vi "Write Driver Config.vi"(8 "error in (no error)":errorcluster, 10 "Driver Config":T1={"Joystick"=refnum, "Forward Drive"=refnum, "Sideways Drive"=refnum, "Percent Forward"=1.0, "Percent Sideways"=1.0}, 11 "Driver in":refnum<class "Driver.lvclass">) -> (0 "error out":errorcluster, 3 "Driver out":refnum<class "Driver.lvclass">)   [LabVIEW 2014, in "Driver.lvlib" / "Driver.lvclass"]
uses:
  Driver.lvclass
  Driver Config.ctl
  Joystick/Joystick Class/Joystick.lvclass
  <vilib>/ActorFramework/Message Enqueuer/Message Enqueuer.lvclass
  Driver.lvclass/Driver.ctl
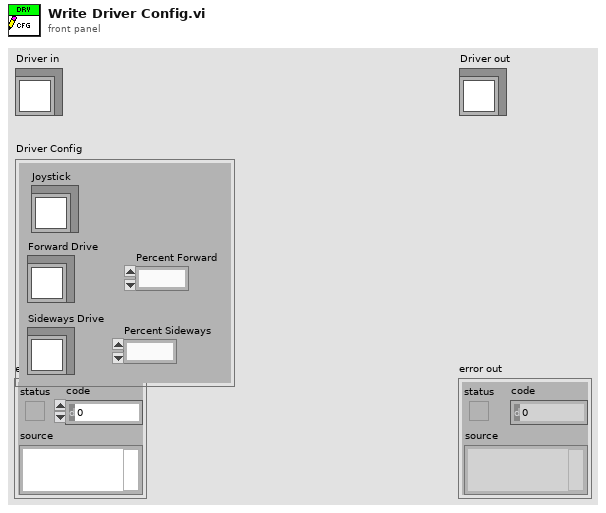
[diagram p1: front panel]
types:
  T1 = typedef "Driver.lvlib/Driver.lvclass/Driver Config.ctl" = cluster{"Joystick":refnum<class "Joystick.lvclass">, "Forward Drive":refnum<class "Message Enqueuer.lvclass">, "Sideways Drive":refnum<class "Message Enqueuer.lvclass">, "Percent Forward":dbl, "Percent Sideways":dbl}
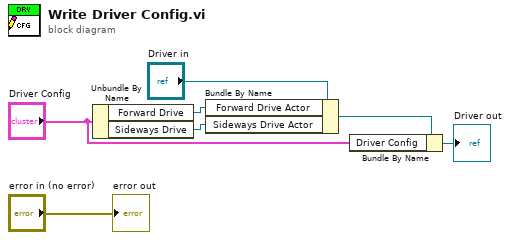
[diagram p0: block diagram]
diagram:
  n1 = Unbundle By Name("Driver Config") -> ("Forward Drive"=w2:refnum<class "Message Enqueuer.lvclass">, "Sideways Drive"=w1:refnum<class "Message Enqueuer.lvclass">)
  n2 = Bundle By Name(cluster="Driver in", "Forward Drive Actor"=w2, "Sideways Drive Actor"=w1) -> (w3:refnum<class "Driver.lvclass">)
  n3 = Bundle By Name(cluster=w3, "Driver Config"="Driver Config") -> (→"Driver out":refnum<class "Driver.lvclass">)
  "error out" <- "error in (no error)"
